vi "_Set Measurement Scale.vi"(6 "Log Scale (dB)":dbl=10.0 min=0.1 max=10.0 step=0.1 format="%.1f", 7 "Reference Level (dBm)":dbl=-10.0 min=-90.0 max=30.0 step=0.1 format="%.1f", 8 "error in (no error)":errorcluster, 9 "Span (nm)":dbl=1100.0 min=0.0 max=2250.0 step=0.5 format="%.3f", 10 "Center (nm)":dbl=1150.0 min=50.0 max=1700.0 step=0.5 format="%.3f", 11 "Yokogawa AQ6370D in":refnum<class "Yokogawa AQ6370D.lvclass">) -> (0 "error out":errorcluster, 3 "Yokogawa AQ6370D out":refnum<class "Yokogawa AQ6370D.lvclass">)   [LabVIEW 2018, in "Yokogawa AQ6370D.lvlib" / "Yokogawa AQ6370D.lvclass"]
uses:
  Yokogawa AQ6370D.lvclass
  Yokogawa AQ6370D.lvclass/Yokogawa AQ6370D.ctl
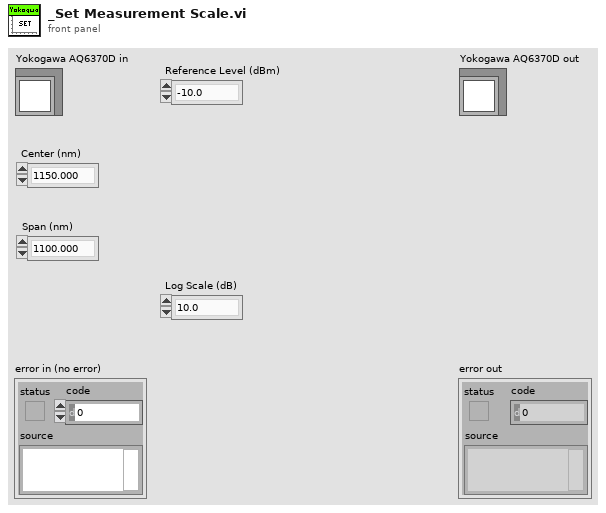
[diagram p1: front panel]
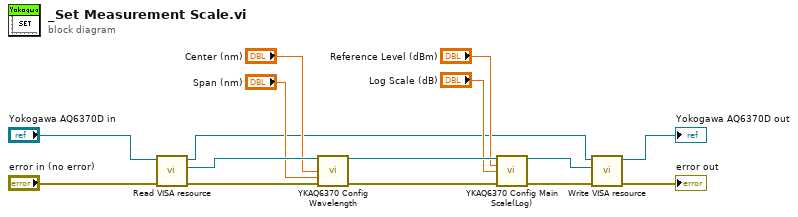
[diagram p0: block diagram]
diagram:
  n1 = call "Read VISA resource.vi"("error in (no error)"="error in (no error)", "Yokogawa AQ6370D in"="Yokogawa AQ6370D in") -> ("error out"=w11:errorcluster, "VISA resource"=w10:refnum<visa-resource-name>, "Yokogawa AQ6370D out"=w5:refnum<class "Yokogawa AQ6370D.lvclass">)  [unwired: 7 in]
  n2 = call <instrlib>:"YKAQ6370 Config Wavelength.vi"("VISA resource name"=w10, "Center/Start (1150.000)"="Center (nm)", "Span/Stop  (1100.000)"="Span (nm)", "error in (no error)"=w11) -> ("VISA resource name out"=w14:refnum<visa-resource-name>, "error out"=w15:errorcluster)  [unwired: 10 in]
  n3 = call <instrlib>:"YKAQ6370 Config Main Scale(Log).vi"("VISA resource name"=w14, "Reference Level (-10.0)"="Reference Level (dBm)", "Log Scale (10.0)"="Log Scale (dB)", "error in (no error)"=w15) -> ("VISA resource name out"=w1:refnum<visa-resource-name>, "error out"=w3:errorcluster)  [unwired: 10 in]
  n4 = call "Write VISA resource.vi"("error in (no error)"=w3, "VISA resource"=w1, "Yokogawa AQ6370D in"=w5) -> ("error out"=→"error out":errorcluster, "Yokogawa AQ6370D out"=→"Yokogawa AQ6370D out":refnum<class "Yokogawa AQ6370D.lvclass">)  [unwired: 7 in]
